vi "ReadCamInterface.vi"(8 "error in (no error)":errorcluster, 11 "ConfigRef In":T1) -> (0 "error out":errorcluster, 3 "ConfigRef Out":T1, 5 "COMPort":refnum<visa-resource-name>)   [LabVIEW 2013]
uses:
  <vilib>/Utility/config.llb/Config Data RefNum.ctl
  <vilib>/Utility/config.llb/Read Key (String).vi
  <vilib>/Utility/config.llb/NI_LVConfig.lvlib
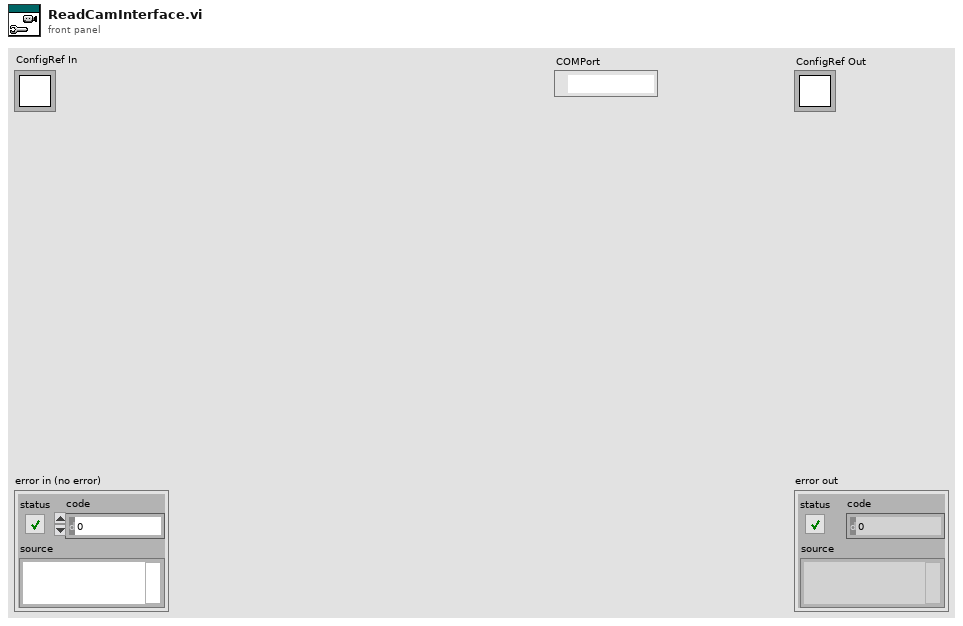
[diagram p1: front panel]
types:
  T1 = typedef "NI_LVConfig.lvlib/Config Data RefNum.ctl" = refnum<k1>
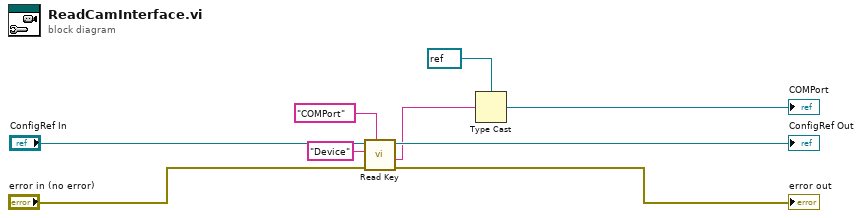
[diagram p0: block diagram]
diagram:
  n1 = call-poly <vilib>:"Read Key.vi"("section"="COMPort", "error in (no error)"="error in (no error)", "key"="Device", "refnum"="ConfigRef In") -> ("error out"=→"error out":errorcluster, "value"=w7:string, "refnum out"=→"ConfigRef Out":T1)  [unwired: 4 in, 1 out]
  n2 = Type Cast(type=refnum<visa-resource-name> refnum ("VISA resource name"), x=w7) -> (*(type *) &x=→"COMPort":refnum<visa-resource-name>)
